vi "Apex controller loop error handler.vi"(8 "error in":errorcluster) -> (0 "error out":errorcluster)   [LabVIEW 2018]
doc: "Handles controller loop errors. This should pretty much never happen since there's very little actual processing done in the controller loop of the kind that can error out. Nearly every case should just be enqueueing commands to the model loop message handler."
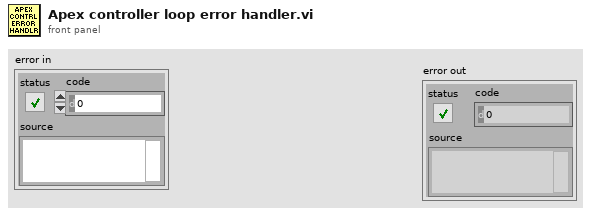
[diagram p1: front panel]
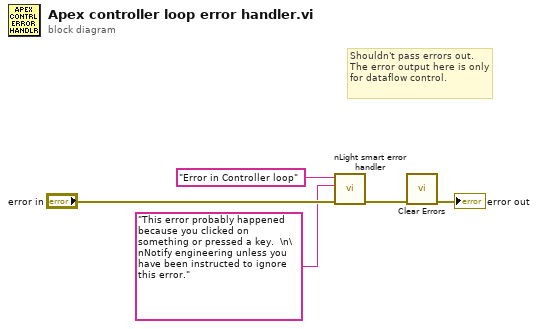
[diagram p0: block diagram]
diagram:
  # "Shouldn't pass errors out.  The error output here is only for dataflow control."
  n1 = call <userlib>:"nLight smart error handler.vi"("error in (no error)"="error in", "Popup message if not in table (Generic message)"="This error probably happened because you clicked on something or pressed a key.  \n\nNotify engineering unless you have been instructed to ignore this error.", "Error title if not in table [<40 chars] (\"LabVIEW error\")"="Error in Controller loop" ("Error title if not in table [<40 chars] (\"LabVIEW error\")")) -> ("error out"=w1:errorcluster)  [unwired: 6 in, 2 out]
  n2 = call <vilib>:"Clear Errors.vi"("error in (no error)"=w1) -> ("error out"=→"error out":errorcluster)  [unwired: 5 in, 1 out]
